vi "Variable_Open Compilation.vi"(0 "scripts manager in":refnum<class "scripts manager.lvclass">, 5 "function in":refnum<class "functionbase.lvclass">, 7 "Variables Name":string[](array[string]), 9 "Variables Value":string[](array[string]), 11 "error in (no error)":errorcluster) -> (4 "scripts manager out":refnum<class "scripts manager.lvclass">, 6 "function":refnum<class "functionbase.lvclass">, 8 "Compilation passed?":bool, 15 "error out":errorcluster)   [LabVIEW 2016, in "scripts manager.lvclass"]
uses:
  scripts manager.lvclass
  functions/functionsbase/functionbase.lvclass
  functions/functionsbase/functionbase.lvclass/functionbase.ctl
  common/variable utils/Valuetype.ctl
  functions/functionsbase/properties/Read Line#.vi
  functions/functionsbase/properties/Read Indent#.vi
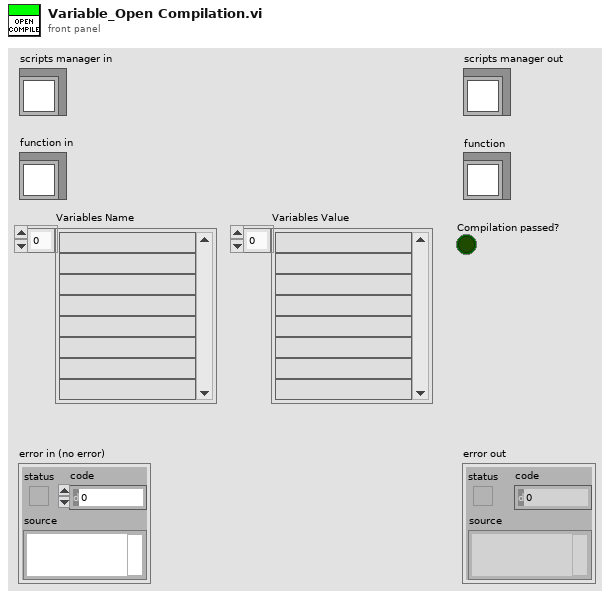
[diagram p1: front panel]
types:
  T1 = typedef "Valuetype.ctl" = enum16{"Value", "Variable", "Function"}
  T2 = typedef "Datatype.ctl" = enum16{"Null", "Numeric", "String", "Bool", "Numeric 1D", "String 1D", "Bool 1D", "Numeric 2D", "String 2D", "Bool 2D", "Variant"}
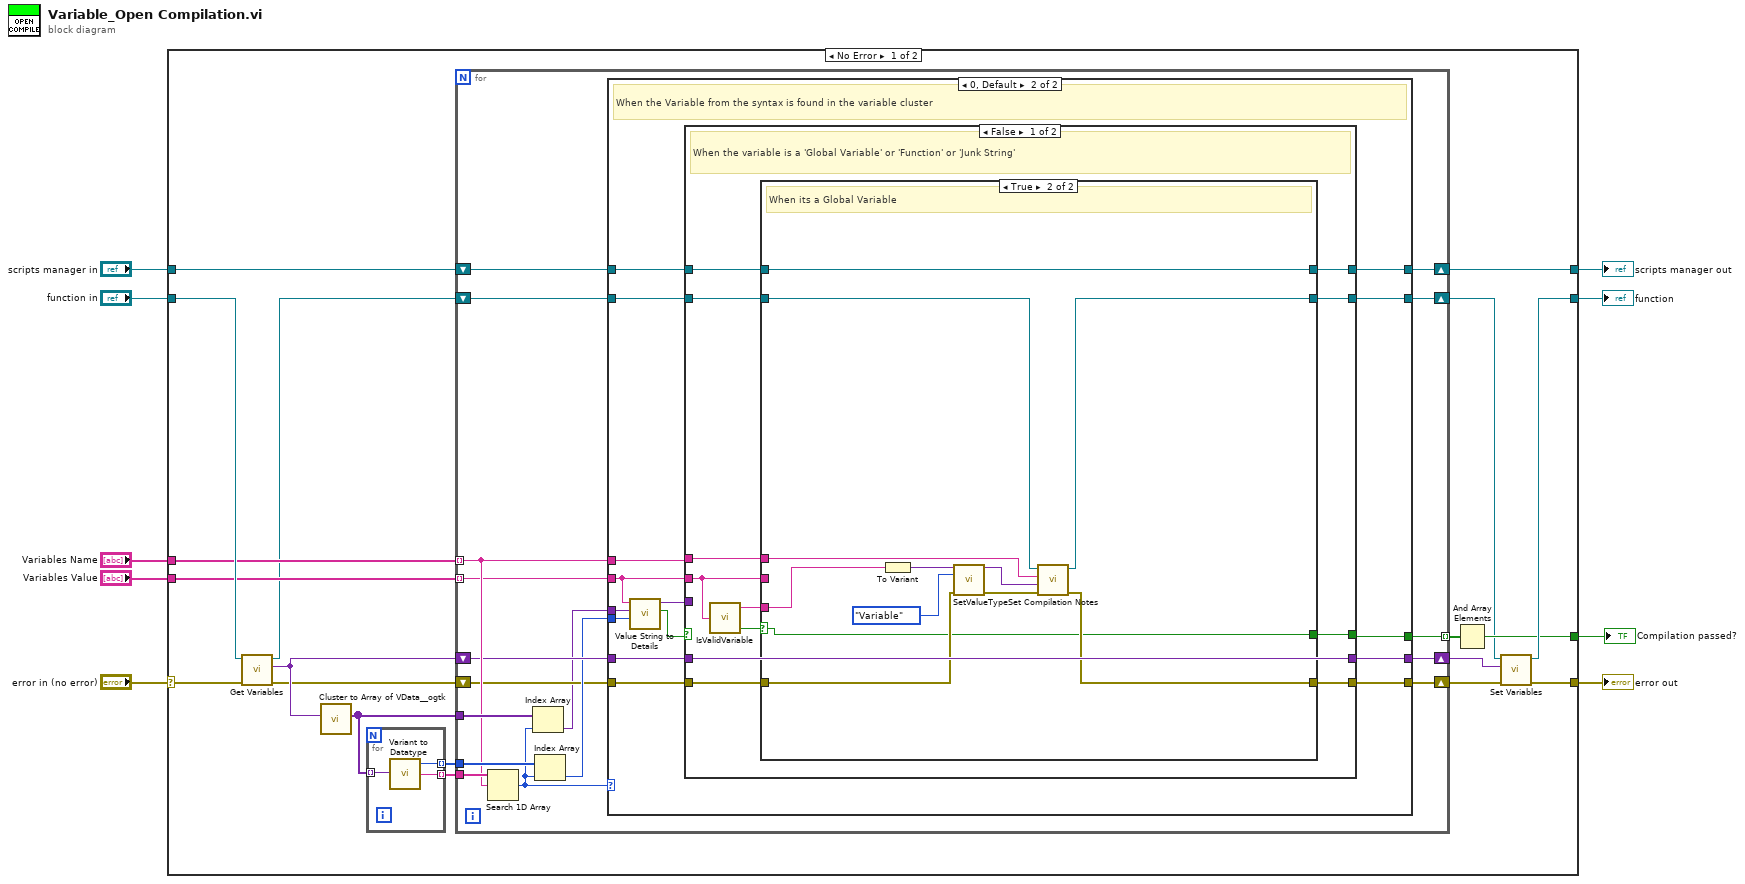
[diagram p0: block diagram]
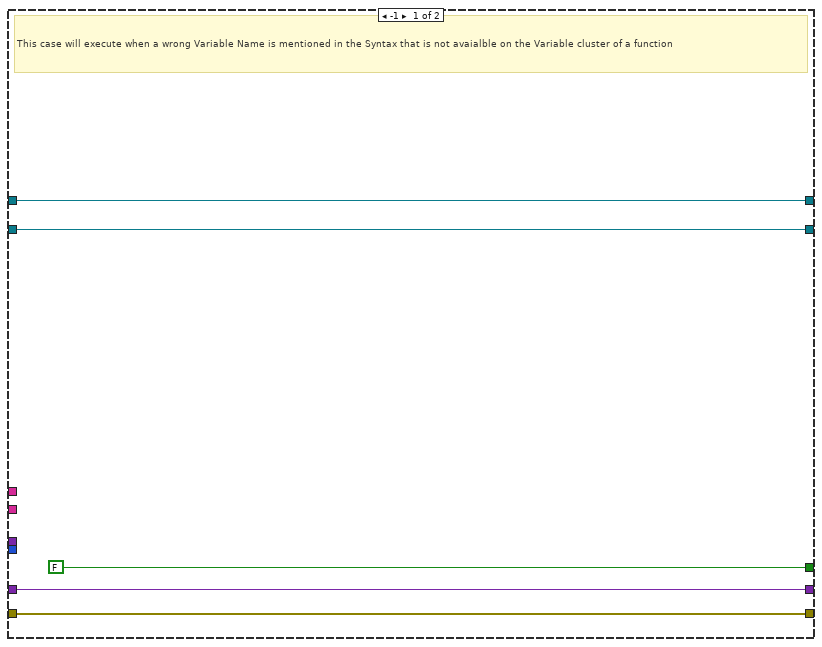
[diagram p2: hidden frame]
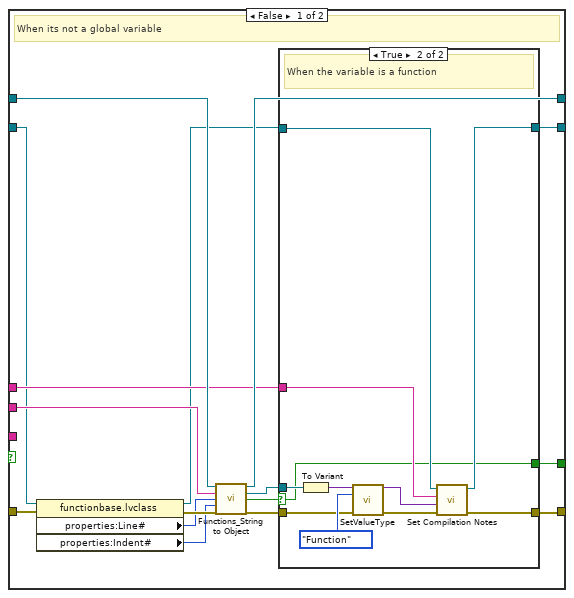
[diagram p3: hidden frame]
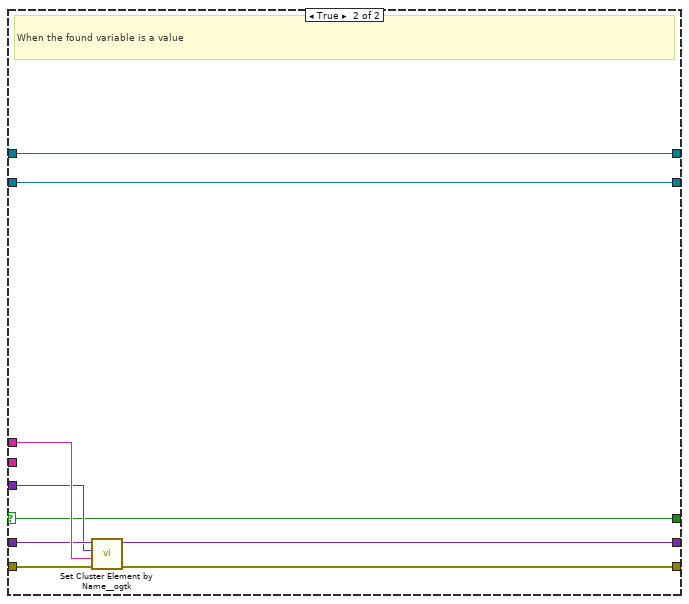
[diagram p5: hidden frame]
diagram:
  n1 = case shown="No Error" "error in (no error)" {
    selector: "error in (no error)" -> [w27 w133]
    tunnel: [w25 w133] -> w8
    tunnel: [w16 w132] -> w6
    tunnel: "scripts manager in" -> [w17 w132]
    tunnel: "function in" -> [w28 _]
    tunnel: [w26 _] -> w4
    tunnel: "Variables Name" -> [w21 _]
    tunnel: "Variables Value" -> [w20 _]
    tunnel: [w12 _] -> w1
    frame No Error {
      n2 = call-dynamic "Get Variables.vi"("error in (no error)"=w27, "functionbase in"=w28) -> ("error out"=w18:errorcluster, "Variables"=w19:variant, "functionbase out"=w11:refnum<class "functionbase.lvclass">)  [unwired: 7 in]
      n3 = call <userlib>:"Cluster to Array of VData__ogtk.vi"("Cluster"=w19) -> ("Array of VData"=w24:variant[])  [unwired: 9 in, 1 out]
      n4 = for {
        tunnel: w24 -> [w131] mode=indexing
        tunnel: [w130] -> w23 mode=indexing
        tunnel: [w129] -> w22 mode=indexing
        n5 = call "Variant to Datatype.vi"("Variant"=w131) -> ("Name"=w129:string, "Datatype"=w130:T2)  [unwired: 2 in, 1 out]
      }
      n6 = for {
        shift-right: [w41] -> w14
        shift-left: w19 -> [w40]
        shift-right: [w39] -> w15
        shift-left: w18 -> [w36]
        tunnel: w24 -> [w43]
        tunnel: w23 -> [w44]
        tunnel: w22 -> [w45]
        tunnel: w21 -> [w42] mode=indexing
        tunnel: w20 -> [w37] mode=indexing
        shift-right: [w29] -> w16
        shift-left: w17 -> [w30]
        tunnel: [w35] -> w13 mode=indexing
        shift-right: [w32] -> w10
        shift-left: w11 -> [w31]
        n7 = Search 1D Array(1D array=w45, element=w42) -> (index of element=w34:i32)  [unwired: 1 in]
        n8 = Index Array(array=w43, index=w34) -> (element=w33:variant)
        n9 = Index Array(array=w44, index=w34) -> (element=w38:T2)
        n10 = case shown="0, Default" w34 {
          tunnel: w42 -> [_ w65]
          tunnel: [w49 w64] -> w41
          tunnel: w40 -> [w49 w63]
          tunnel: [w50 w62] -> w39
          tunnel: w38 -> [_ w61]
          tunnel: w37 -> [_ w55]
          tunnel: w36 -> [w50 w60]
          tunnel: [FALSE w57] -> w35
          tunnel: w33 -> [_ w56]
          tunnel: [w47 w54] -> w32
          tunnel: w31 -> [w47 w53]
          tunnel: w30 -> [w46 w52]
          tunnel: [w46 w51] -> w29
          frame -1 {
            # "This case will execute when a wrong Variable Name is mentioned in the Syntax that is not avaialble on the Variable cluster of a function"
          }
          frame 0, Default {
            # "When the Variable from the syntax is found in the variable cluster"
            n11 = call "Value String to Details.vi"("Datatype"=w61, "Default"=w56, "Value String"=w55) -> ("Identified?"=w58:bool, "Value Variant"=w59:variant)  [unwired: 7 in]
            n12 = case shown="False" w58 {
              selector: w58 -> [_ w122]
              tunnel: w65 -> [w75 w128]
              tunnel: [w77 w127] -> w64
              tunnel: w63 -> [w77 w126]
              tunnel: [w74 w125] -> w62
              tunnel: w60 -> [w72 w124]
              tunnel: w59 -> [_ w123]
              tunnel: [w66 w122] -> w57
              tunnel: w55 -> [w67 _]
              tunnel: [w71 w121] -> w54
              tunnel: w53 -> [w76 w121]
              tunnel: w52 -> [w69 w120]
              tunnel: [w68 w120] -> w51
              frame False {
                # "When the variable is a 'Global Variable' or 'Function' or 'Junk String'"
                n13 = call "IsValidVariable.vi"("Value String in"=w67) -> ("IsVariable"=w70:bool, "Variable Name"=w73:string)  [unwired: 3 in]
                n14 = case shown="True" w70 {
                  selector: w70 -> [_ w108]
                  tunnel: w76 -> [w79 w119]
                  tunnel: w75 -> [w88 w118]
                  tunnel: [w86 w117] -> w74
                  tunnel: w73 -> [_ w115]
                  tunnel: w72 -> [w83 w111]
                  tunnel: [w87 w110] -> w71
                  tunnel: w69 -> [w93 w109]
                  tunnel: [w91 w109] -> w68
                  tunnel: w67 -> [w92 _]
                  tunnel: [w84 w108] -> w66
                  frame False {
                    # "When its not a global variable"
                    n15 = property class="functionbase.lvclass"(reference=w79, error in=w83) -> (reference out=w78:refnum<class "functionbase.lvclass">, error out=w82:errorcluster, "properties:Line#"=w81:i64, "properties:Indent#"=w80:i64)
                    n16 = call-dynamic "Functions_String to Object.vi"("scripts manager in"=w93, "Functions"=w92, "Line#"=w81, "Indent#"=w80, "error in (no error)"=w82) -> ("scripts manager out"=w91:refnum<class "scripts manager.lvclass">, "function obj"=w90:refnum<class "functionbase.lvclass">, "function created"=w85:bool, "error out"=w89:errorcluster)  [unwired: 7 in]
                    n17 = case shown="True" w85 {
                      selector: w85 -> [w94 w97]
                      tunnel: w90 -> [_ w103]
                      tunnel: w89 -> [w95 w102]
                      tunnel: w88 -> [_ w101]
                      tunnel: w78 -> [w96 w100]
                      tunnel: [w96 w99] -> w87
                      tunnel: [w95 w98] -> w86
                      tunnel: [w94 w97] -> w84
                      frame False {
                        # "When its not a function"
                      }
                      frame True {
                        # "When the variable is a function"
                        n18 = To Variant(anything=w103) -> (Variant=w106:variant)
                        n19 = call "SetValueType.vi"("variant"=w106, "valuetype"=Valuetype."Function", "error in"=w102) -> ("variant out"=w105:variant, "error out"=w104:errorcluster)  [unwired: 11 in]
                        n20 = call "Set Compilation Notes.vi"("error in (no error)"=w104, "Notes"=w105, "note key"=w101, "functionbase in"=w100) -> ("error out"=w98:errorcluster, "functionbase out"=w99:refnum<class "functionbase.lvclass">)  [unwired: 6 in]
                      }
                    }
                  }
                  frame True {
                    # "When its a Global Variable"
                    n21 = To Variant(anything=w115) -> (Variant=w114:variant)
                    n22 = call "SetValueType.vi"("variant"=w114, "valuetype"=Valuetype."Variable", "error in"=w111) -> ("variant out"=w113:variant, "error out"=w112:errorcluster)  [unwired: 11 in]
                    n23 = call "Set Compilation Notes.vi"("error in (no error)"=w112, "Notes"=w113, "note key"=w118, "functionbase in"=w119) -> ("error out"=w117:errorcluster, "functionbase out"=w110:refnum<class "functionbase.lvclass">)  [unwired: 6 in]
                  }
                }
              }
              frame True {
                # "When the found variable is a value"
                n24 = call <userlib>:"Set Cluster Element by Name__ogtk.vi"("error in (no error)"=w124, "Element Name (\"\": New Element Data Name)"=w128, "New Element Value"=w123, "Cluster"=w126) -> ("error out"=w125:errorcluster, "VCluster out"=w127:variant)  [unwired: 5 in, 1 out]
              }
            }
          }
        }
      }
      n25 = And Array Elements(Boolean array=w13) -> (logical AND=w12:bool)
      n26 = call-dynamic "Set Variables.vi"("error in (no error)"=w15, "Variables"=w14, "functionbase in"=w10) -> ("error out"=w25:errorcluster, "functionbase out"=w26:refnum<class "functionbase.lvclass">)  [unwired: 7 in]
    }
    frame Error {
    }
  }
  "error out" <- w8
  "scripts manager out" <- w6
  "function" <- w4
  "Compilation passed?" <- w1
